vi "Remove Duplicates from 1D Array__ogtk.vi"   [LabVIEW 2016]
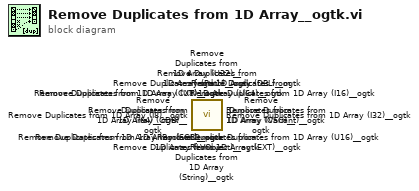
[diagram p0: block diagram]
diagram:
  n1 = call <userlib>:"Remove Duplicates from 1D Array (LVObject)__ogtk.vi"() -> ()  [unwired: 1 in, 2 out]
  n2 = call <userlib>:"Remove Duplicates from 1D Array (U64)__ogtk.vi"() -> ()  [unwired: 1 in, 2 out]
  n3 = call <userlib>:"Remove Duplicates from 1D Array (I64)__ogtk.vi"() -> ()  [unwired: 1 in, 2 out]
  n4 = call <userlib>:"Remove Duplicates from 1D Array (Variant)__ogtk.vi"() -> ()  [unwired: 1 in, 2 out]
  n5 = call <userlib>:"Remove Duplicates from 1D Array (U8)__ogtk.vi"() -> ()  [unwired: 1 in, 2 out]
  n6 = call <userlib>:"Remove Duplicates from 1D Array (U32)__ogtk.vi"() -> ()  [unwired: 1 in, 2 out]
  n7 = call <userlib>:"Remove Duplicates from 1D Array (U16)__ogtk.vi"() -> ()  [unwired: 1 in, 2 out]
  n8 = call <userlib>:"Remove Duplicates from 1D Array (String)__ogtk.vi"() -> ()  [unwired: 1 in, 2 out]
  n9 = call <userlib>:"Remove Duplicates from 1D Array (SGL)__ogtk.vi"() -> ()  [unwired: 1 in, 2 out]
  n10 = call <userlib>:"Remove Duplicates from 1D Array (I8)__ogtk.vi"() -> ()  [unwired: 1 in, 2 out]
  n11 = call <userlib>:"Remove Duplicates from 1D Array (I32)__ogtk.vi"() -> ()  [unwired: 1 in, 2 out]
  n12 = call <userlib>:"Remove Duplicates from 1D Array (I16)__ogtk.vi"() -> ()  [unwired: 1 in, 2 out]
  n13 = call <userlib>:"Remove Duplicates from 1D Array (EXT)__ogtk.vi"() -> ()  [unwired: 1 in, 2 out]
  n14 = call <userlib>:"Remove Duplicates from 1D Array (DBL)__ogtk.vi"() -> ()  [unwired: 1 in, 2 out]
  n15 = call <userlib>:"Remove Duplicates from 1D Array (CXT)__ogtk.vi"() -> ()  [unwired: 1 in, 2 out]
  n16 = call <userlib>:"Remove Duplicates from 1D Array (CSG)__ogtk.vi"() -> ()  [unwired: 1 in, 2 out]
  n17 = call <userlib>:"Remove Duplicates from 1D Array (CDB)__ogtk.vi"() -> ()  [unwired: 1 in, 2 out]
  n18 = call <userlib>:"Remove Duplicates from 1D Array (Path)__ogtk.vi"() -> ()  [unwired: 1 in, 2 out]
  n19 = call <userlib>:"Remove Duplicates from 1D Array (Boolean)__ogtk.vi"() -> ()  [unwired: 1 in, 2 out]
